vi "SwerveOdometry_UpdateX.vi"(4 "Time":dbl=-1.0 format="%33.4f", 7 "SWERVE_DRIVE_KINEMATICS":T1 {"SavedModuleStates"."Angle"."SIN" format="%13.4f"; "SavedModuleStates"."Angle"."COS" format="%13.4f"; "SavedModuleStates"."Angle"."VALUE" format="%13.4f"; "PrevCoR"."Y" format="%14.3f"; "PrevCoR"."X" format="%14.3f"; "Modules"."Y" format="%14.3f"; "Modules"."X" format="%14.3f"}, 8 "gyroAngle":T5={"VALUE"=0.0, "COS"=1.0, "SIN"=0.0} {"SIN" format="%13.4f"; "COS" format="%13.4f"; "VALUE" format="%13.4f"}, 9 "module States":T4[](array[typedef]) {"Angle"."SIN" format="%13.4f"; "Angle"."COS" format="%13.4f"; "Angle"."VALUE" format="%13.4f"}, 11 "in SWERVE_DRIVE_ODOMETRY":T7={"POSE"={"TRANSLATION"={"X"=0.0, "Y"=0.0}, "ROTATION"={"VALUE"=0.0, "COS"=1.0, "SIN"=0.0}}, "GyroOffset"={"VALUE"=0.0, "COS"=1.0, "SIN"=0.0}, "PreviousAngle"={"VALUE"=0.0, "COS"=1.0, "SIN"=0.0}, "PrevModulePositions"=[], "NumModules"=0} {"PrevModulePositions"."Angle"."SIN" format="%13.4f"; "PrevModulePositions"."Angle"."COS" format="%13.4f"; "PrevModulePositions"."Angle"."VALUE" format="%13.4f"; "PreviousAngle"."SIN" format="%13.4f"; "PreviousAngle"."COS" format="%13.4f"; "PreviousAngle"."VALUE" format="%13.4f"; "GyroOffset"."SIN" format="%13.4f"; "GyroOffset"."COS" format="%13.4f"; "GyroOffset"."VALUE" format="%13.4f"; "POSE"."ROTATION"."SIN" format="%13.4f"; "POSE"."ROTATION"."COS" format="%13.4f"; "POSE"."ROTATION"."VALUE" format="%13.4f"; "POSE"."TRANSLATION"."Y" format="%14.3f"; "POSE"."TRANSLATION"."X" format="%14.3f"}) -> (1 "robot POSE":T6={"TRANSLATION"={"X"=0.0, "Y"=0.0}, "ROTATION"={"VALUE"=0.0, "COS"=1.0, "SIN"=0.0}} {"ROTATION"."SIN" format="%13.4f"; "ROTATION"."COS" format="%13.4f"; "ROTATION"."VALUE" format="%13.4f"; "TRANSLATION"."Y" format="%14.3f"; "TRANSLATION"."X" format="%14.3f"}, 3 "out SWERVE_DRIVE_ODOMETRY":T7={"POSE"={"TRANSLATION"={"X"=0.0, "Y"=0.0}, "ROTATION"={"VALUE"=0.0, "COS"=1.0, "SIN"=0.0}}, "GyroOffset"={"VALUE"=0.0, "COS"=1.0, "SIN"=0.0}, "PreviousAngle"={"VALUE"=0.0, "COS"=1.0, "SIN"=0.0}, "PrevModulePositions"=[], "NumModules"=0} {"PrevModulePositions"."Angle"."SIN" format="%13.4f"; "PrevModulePositions"."Angle"."COS" format="%13.4f"; "PrevModulePositions"."Angle"."VALUE" format="%13.4f"; "PreviousAngle"."SIN" format="%13.4f"; "PreviousAngle"."COS" format="%13.4f"; "PreviousAngle"."VALUE" format="%13.4f"; "GyroOffset"."SIN" format="%13.4f"; "GyroOffset"."COS" format="%13.4f"; "GyroOffset"."VALUE" format="%13.4f"; "POSE"."ROTATION"."SIN" format="%13.4f"; "POSE"."ROTATION"."COS" format="%13.4f"; "POSE"."ROTATION"."VALUE" format="%13.4f"; "POSE"."TRANSLATION"."Y" format="%14.3f"; "POSE"."TRANSLATION"."X" format="%14.3f"})   [LabVIEW 2019]
doc: "Updates the robot's position on the field using forward kinematics and integration of the pose over time. This method automatically calculates the current time to calculate period (difference between two timestamps). The period is used to calculate the change in distance from a velocity. This also takes in an angle parameter which is used instead of the angular rate that is calculated from forward kinematics.\n\nParameters: \n - InSwerveDriveOdometry - This data structure \n - gyroAngle - The angle reported by the gyroscope.\n - moduleStates - The current state of all swerve modules. Please provide the states in the same order in which you instantiated your SwerveDriveKinematics.\n\nReturns:\n - OutSwerveDriveOdometry - Updated data structure\n - robot pose - The new pose of the robot."
uses:
  Trajectory_Library.lvlib
  TypeDef/TRANSLATION2D.ctl
  TypeDef/ROTATION2D.ctl
  TypeDef/POSE2D.ctl
  TypeDef/SWERVE_DRIVE_ODOMETRY.ctl
  TypeDef/SWERVE_DRIVE_MODULE_STATE.ctl
  <vilib>/Analysis/Matrix/Datatypes/RealMatrix.ctl
  <vilib>/Analysis/Matrix/NI_Matrix.lvlib
  TypeDef/SWERVE_DRIVE_KINEMATICS.ctl
  TypeDef/SWERVE_DRIVE_MODULE_POSITION.ctl
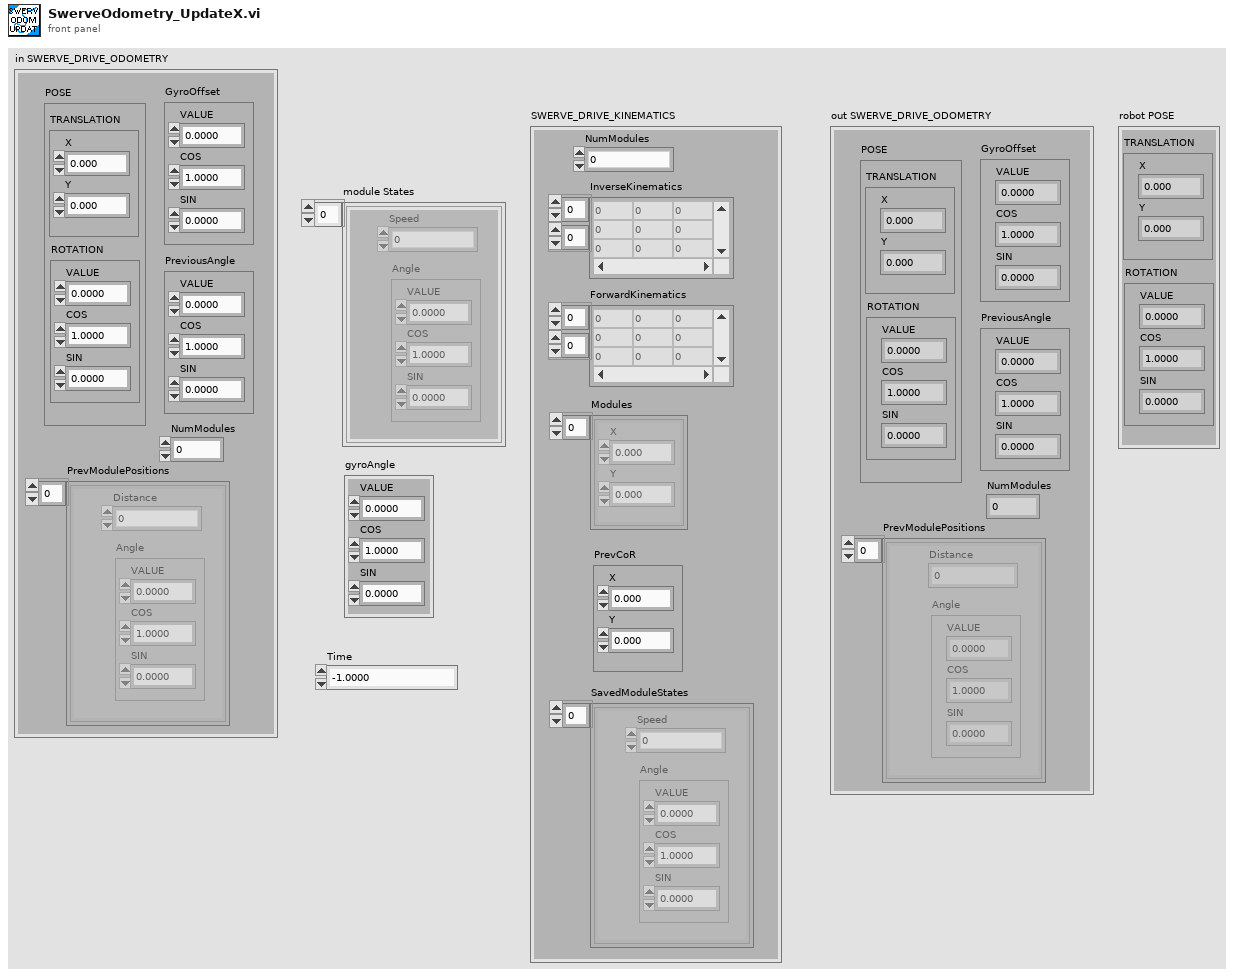
[diagram p1: front panel]
types:
  T1 = typedef "Trajectory_Library.lvlib/SWERVE_DRIVE_KINEMATICS.ctl" = cluster{"NumModules":i32, "InverseKinematics":T2, "ForwardKinematics":T2, "Modules":T3[], "PrevCoR":T3, "SavedModuleStates":T4[]}
  T2 = typedef "NI_Matrix.lvlib/RealMatrix.ctl" = dbl[][]
  T3 = typedef "Trajectory_Library.lvlib/TRANSLATION2D.ctl" = cluster{"X":dbl, "Y":dbl}
  T4 = typedef "Trajectory_Library.lvlib/SWERVE_DRIVE_MODULE_STATE.ctl" = cluster{"Speed":dbl, "Angle":T5}
  T5 = typedef "Trajectory_Library.lvlib/ROTATION2D.ctl" = cluster{"VALUE":dbl, "COS":dbl, "SIN":dbl}
  T6 = typedef "Trajectory_Library.lvlib/POSE2D.ctl" = cluster{"TRANSLATION":T3, "ROTATION":T5}
  T7 = typedef "Trajectory_Library.lvlib/SWERVE_DRIVE_ODOMETRY.ctl" = cluster{"POSE":T6, "GyroOffset":T5, "PreviousAngle":T5, "PrevModulePositions":T8[], "NumModules":i32}
  T8 = typedef "Trajectory_Library.lvlib/SWERVE_DRIVE_MODULE_POSITION.ctl" = cluster{"Distance":dbl, "Angle":T5}
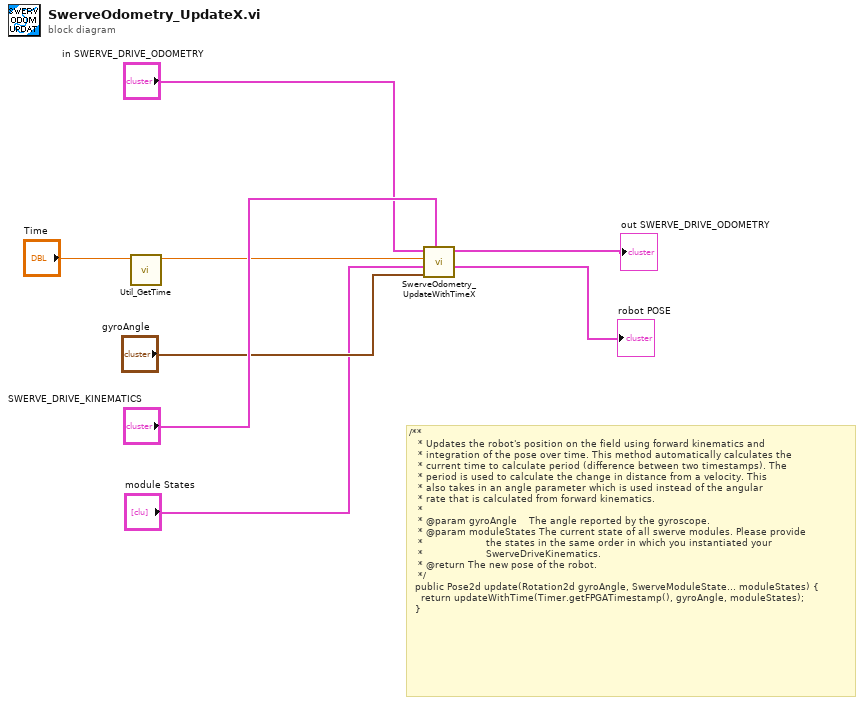
[diagram p0: block diagram]
diagram:
  # "/**\n   * Updates the robot's position on the field using forward kinematics and\n   * integration of the pose over time. This method automatically calculates the\n   * current time to calculate period (difference between two timestamps). The\n   * period is used to calculate the change in distance from a velocity. This\n   * also takes in an angle parameter which is used instead of the angular\n   * rate that is calculated from forward kinematics.\n   *\n   * @param gyroAngle    The angle reported by the gyroscope.\n   * @param moduleStates The current state of all swerve modules. Please provide\n   *                     the states in the same order in which you instantiated your\n   *                     SwerveDriveKinematics.\n   * @return The new pose of the robot.\n   */\n  public Pose2d update(Rotation2d gyroAngle, SwerveModuleState... moduleStates) {\n    return updateWithTime(Timer.getFPGATimestamp(), gyroAngle, moduleStates);\n  }"
  n1 = call "Util_GetTime.vi"("Pass_Through_Time"="Time") -> ("FPGA_Time_Seconds"=w2:dbl)  [unwired: 9 in, 1 out]
  n2 = call "SwerveOdometry_UpdateWithTimeX.vi"("SWERVE_DRIVE_KINEMATICS"="SWERVE_DRIVE_KINEMATICS", "gyroAngle"="gyroAngle", "module States"="module States", "Time"=w2, "in SWERVE_DRIVE_ODOMETRY"="in SWERVE_DRIVE_ODOMETRY") -> ("robot POSE"=→"robot POSE":T6, "out SWERVE_DRIVE_ODOMETRY"=→"out SWERVE_DRIVE_ODOMETRY":T7)  [unwired: 5 in]
